vi "Protected Enqueue.vi"(8 "error in (no error)":errorcluster, 9 "Data":variant, 10 "Msg":string, 11 "Message Queue in":refnum<class "Message Queue.lvclass">) -> (0 "error out":errorcluster, 3 "Message Queue out":refnum<class "Message Queue.lvclass">)   [LabVIEW 2019, in "Network Interface.lvlib" / "Message Queue.lvclass"]
uses:
  <vilib>/gpm_packages/@cs/Network-Sink/Source/Network Interface/Message Queue/Message Queue.lvclass
  <vilib>/gpm_packages/@cs/Network-Sink/Source/Network Interface/Message Queue/Message Queue.lvclass/Message Queue.ctl
  <vilib>/gpm_packages/@cs/Network-Sink/Source/Network Interface/Message Queue/Message Cluster.ctl
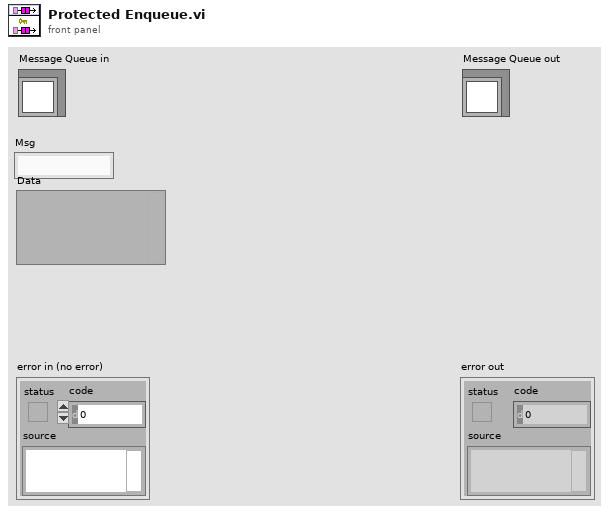
[diagram p1: front panel]
types:
  T1 = typedef "Network Interface.lvlib/Message Queue.lvclass/Message Cluster.ctl" = cluster{"Msg":string, "Data":variant}
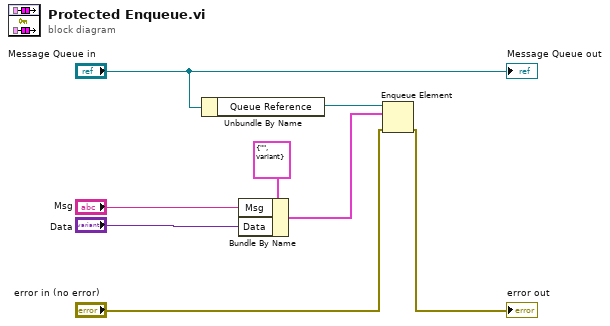
[diagram p0: block diagram]
diagram:
  n1 = Unbundle By Name("Message Queue in") -> ("Queue Reference"=w7:refnum<queue>)
  n2 = Bundle By Name(cluster=T1 {"Msg"="", "Data"=variant} ("element"), "Msg"="Msg", "Data"="Data") -> (w5:T1)
  n3 = Enqueue Element(queue=w7, element=w5, error in (no error)="error in (no error)") -> (error out=→"error out":errorcluster)  [unwired: 1 in, 2 out]
  "Message Queue out" <- "Message Queue in"
